vi "Start.vi"(8 "error in (no error)":errorcluster, 11 "Volatus Core in":refnum<class "Volatus Core.lvclass">) -> (0 "error out":errorcluster, 2 "MessageQ":refnum<class "MessageQ.lvclass">)   [LabVIEW 2020, in "Volatus.lvlib" / "Volatus Core.lvclass"]
uses:
  Volatus Core.lvclass
  C:/dev/lv20CE/relink/lv-volatus/Volatus/Module/Module.lvclass
  MessageQ/MessageQ.lvclass
  VolatusAPI/VolatusAPI.lvclass
  VolatusConfig/VolatusConfigElement/VolatusConfigElement.lvclass
  Volatus Core.lvclass/Volatus Core.ctl
  Module/Module.lvclass
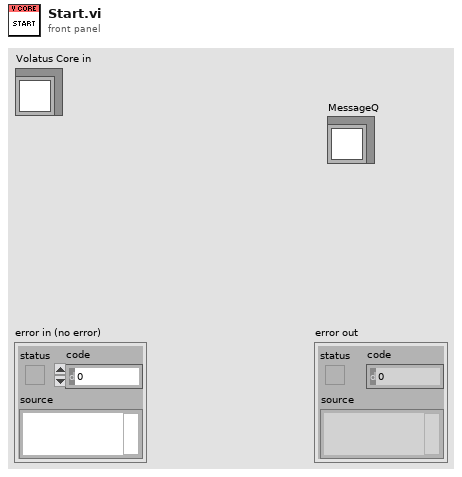
[diagram p1: front panel]
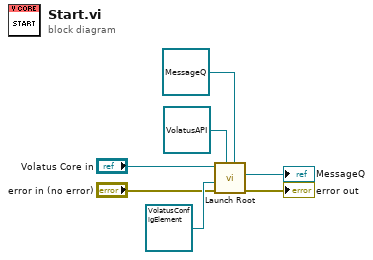
[diagram p0: block diagram]
diagram:
  n1 = call "Launch Root.vi"("Status Q"=refnum<class "MessageQ.lvclass"> refnum, "VolatusAPI"=refnum<class "VolatusAPI.lvclass"> refnum, "error in (no error)"="error in (no error)", "Config Element"=refnum<class "VolatusConfigElement.lvclass"> refnum, "Module in"="Volatus Core in") -> ("error out"=→"error out":errorcluster, "MessageQ"=→"MessageQ":refnum<class "MessageQ.lvclass">)  [unwired: 5 in]
